vi "NF87XX.set start velocity.vi"(0 "i ref in":refnum<vi>, 1 "System":string="N/A", 2 "start velocity (0 .. 1999)":dbl min=0.0 max=1999.0, 3 "Motor (0,1,2)":i32, 5 "error in (no error)":errorcluster) -> (14 "i ref out":refnum<vi>, 19 "error out":errorcluster)   [LabVIEW 2014, in "NF87XX.lvlib"]
doc: "Sets the start velocity for the motor which must be 0, 1 or 2. The start velocity [steps/s] is coerced to the allowed range of 0 ... 1999.\n\nauthor: Stefan Götte\ndata: 09-JAN-2007\n\n\nLicense Agreement for this software:\n\nCopyright (C)\nGesellschaft für Schwerionenforschung, GSI\nPlanckstr. 1\n64291 Darmstadt\nGermany\n\nContact: D.Beck@gsi.de \n\nThis program is free software; you can redistribute it and/or modify it under the terms of the GNU General Public License as published by the Free Software Foundation; either version 2 of the license, or (at your option) any later version.\n\nThis program is distributed in the hope that it will be useful, but WITHOUT ANY WARRANTY; without even the implied warranty of MERCHANTABILITY or FITNESS FOR A PARTICULAR PURPOSE. See the GNU General License for more details (http://www.gnu.org).\n\nGesellschaft für Schwerionenforschung, GSI\nPlanckstr. 1, 64291 Darmstadt, Germany\nFor all questions and ideas contact: M.Richter@gsi.de, H.Brand@gsi.de or D.Beck@gsi.de.\nLast update: 17-JUN-2004"
uses:
  NF87XX.lvlib
  instr.lib/NewFocusPico/Pico Parameters.ctl
  CS_Core/CSSystem/CoreDefs/CoreDefs.error_type.ctl
  CS_Core/CSSystem/CoreLib/CoreLib.lvlib
  instr.lib/NewFocusPico/NewFocusPico - Driver np.lvlib
panel:
  in  "Pico Parameter type":T1={"Pico Type"=enum."Open-Loop Pico", "Acceleration (steps/sec^2)"="32000", "Velocity ( Hz)"="2000", "Driver"="A1", "Motor"="0", "Channel"="0", "Process Step"=""}
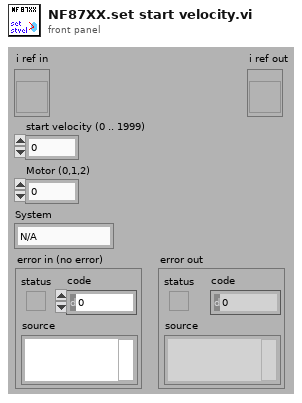
[diagram p1: front panel]
types:
  T1 = typedef "NewFocusPico - Driver np.lvlib/Pico Parameters.ctl" = cluster{"Pico Type":enum16{"Open-Loop Pico", "Close-Loop Pico", "Pico Ultra"}, "Acceleration (steps/sec^2)":string, "Velocity ( Hz)":string, "Driver":string, "Motor":string, "Channel":string, "Process Step":string}
  T2 = typedef "NF87XX.lvlib/NF87XX.driver Type.ctl" = enum16{"not defined", "3-ch open loop drv", "1-ch closed loop drv"}
  T3 = typedef "CoreDefs.error_type.ctl" = enum16{"no error", "can't load process", "can't unload process", "process does not exist", "can't install process", "can't remove process", "unknown function", "time out", "can't execute function", "duplicate queue name", "super not found", "caller queue invalid", "can't ping process", "unknown error", "VISA Error", "VISA timeout", "GPIB timeout", "GPIB error", "communication error", "data type mismatch", "can't read data from OPC server", "can't write data to OPC server", "OET error", "function not implemented", "process already exists", "invalid Shared Variable name", "error writing Shared Variable", "error reading Shared Variable", "invalid client name", "corrupt database", "unknown class", "call not authorized", "parameter out of range", "OET timeout: can't get data to modify", "invalid queue name", "requested operation incompatible with current state", "event undefined", "event disabled", "state undefined", "caller is not a friend", "EventBuilder: bad eventID", "EventBuilder: no DAQ devices", "a thread must not stop itself", "UNUSED ELEMENT4", "DiscArchiver: eventData incomplete", "DiscArchiver: eventData does not belong to run", "DiscArchiver: can't open file", "DiscArchiver: can't write to file", "DiscArchiver: available disc space low", "can't acquire semaphore", "error reading data from database", "notifier object is not existing", "can't register process", "can't unregister process", "illegal event type", "object disabled", "object already exists", "can't change state", "Instrument not found", "no connection to remote node", "invalid reference", "N/A", "UNUSED ELEMENT 1", "element not found", "illegal TCP/IP connection detected", "object does not exist", "invalid access ID", "unknown CS system", "invalid privilige", "unsupported data type", "unsupported server type", "IO server already exists", "Shared Variable already exists"}
  T4 = enum16{"User....", "DEF", "DIAG", "INI", "LOCK", "UNLOCK", "MAP", "SAV", "VER", "ACC", "CHL", "FOR", "GO", "HAL", "MOF", "MON", "MPV", "POS", "REL", "REV", "STA", "STO", "TYP", "VEL", "ABS", "SER", "NOS", "DRT", "FLI", "RLI", "FIN", "RIN", "AIN", "IN", "JOF", "JON", "OUT", "RES FINE", "RES COARSE", "02 (HEX)", "PWM", "CNT", "TMR", "HOSTNAME", "IPADDR", "IPMODE", "NETMASK", "GATEWAY", "DNSSRVR", "PASSWD", "ECHO", "MACADDR"}
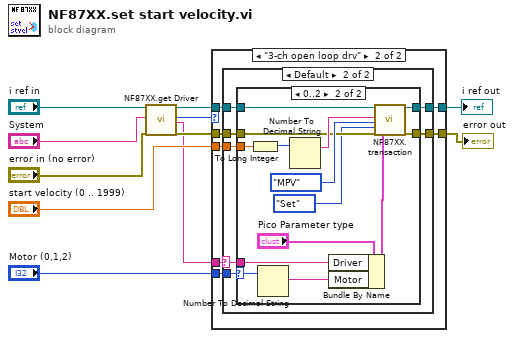
[diagram p0: block diagram]
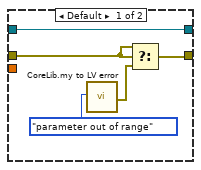
[diagram p4: hidden frame]
diagram:
  n1 = call "NF87XX.get Driver.vi"("i ref in"="i ref in", "System"="System", "error in (no error)"="error in (no error)") -> ("i ref out"=w4:refnum<vi>, "Driver Type"=w1:T2, "Driver"=w2:string, "error out"=w3:errorcluster)  [unwired: 12 in, 1 out]
  n2 = case shown="\"3-ch open loop drv\"" w1 {
    tunnel: "Motor (0,1,2)" -> [_ w20]
    tunnel: "start velocity (0 .. 1999)" -> [_ w19]
    tunnel: [w13 w18] -> w6
    tunnel: [w12 w17] -> w5
    tunnel: w4 -> [w13 w16]
    tunnel: w3 -> [w12 w15]
    tunnel: w2 -> [_ w14]
    frame "not defined", Default {
    }
    frame "3-ch open loop drv" {
      n3 = case shown="Default" w14 {
        selector: w14 -> [_ w23]
        tunnel: [w22 w29] -> w18
        tunnel: [w21 w28] -> w17
        tunnel: w19 -> [_ w27]
        tunnel: w20 -> [_ w26]
        tunnel: w16 -> [w22 w25]
        tunnel: w15 -> [w21 w24]
        frame "N/A" {
        }
        frame Default {
          n4 = case shown="0..2" w26 {
            selector: w26 -> [_ w39]
            tunnel: [w34 w48] -> w29
            tunnel: [w30 w47] -> w28
            tunnel: w25 -> [w34 w38]
            tunnel: w27 -> [_ w46]
            tunnel: w24 -> [w31 w37]
            tunnel: w23 -> [_ w36]
            frame Default {
              n5 = call "CoreLib.my to LV error.vi"("ErrorTypes"=CoreDefs.error_type."parameter out of range") -> ("myErrorCluster"=w33:errorcluster)  [unwired: 17 in, 1 out]
              n6 = Select(t=w31, s=w31, f=w33) -> (s? t:f=w30:errorcluster)
            }
            frame 0..2 {
              n7 = To Long Integer(number=w46) -> (32bit integer=w45:i32)
              n8 = Number To Decimal String(number=w39) -> (decimal integer string=w41:string)  [unwired: 1 in]
              n9 = Number To Decimal String(number=w45) -> (decimal integer string=w44:string)  [unwired: 1 in]
              n10 = Bundle By Name(cluster="Pico Parameter type", "Driver"=w36, "Motor"=w41) -> (w40:T1)
              n11 = call "NF87XX.transaction.vi"("i ref in"=w38, "User Cmd/Numeric Argu"=w44, "MCL Cmd"=T4."MPV", "Query/Set"=enum16{"Query", "Set"}."Set", "error in (no error)"=w37, "Pico Parameter"=w40) -> ("i ref out"=w48:refnum<vi>, "error out"=w47:errorcluster)  [unwired: 11 in, 1 out]
            }
          }
        }
      }
    }
  }
  "error out" <- w5
  "i ref out" <- w6
